vi "pulse.vi"(4 "error in":errorcluster, 5 "dwell after":u32, 6 "time on":u32, 7 "lines 2":tag) -> (0 "error out":errorcluster)   [LabVIEW 2012]
panel:
  in  "stop":bool
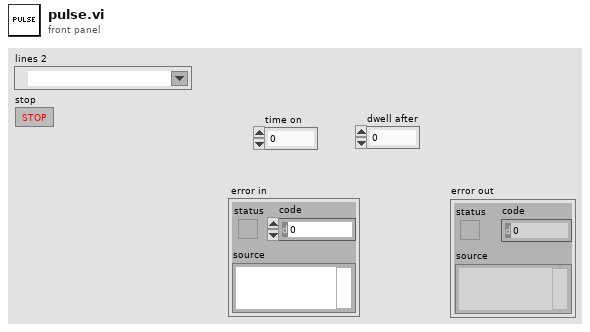
[diagram p1: front panel]
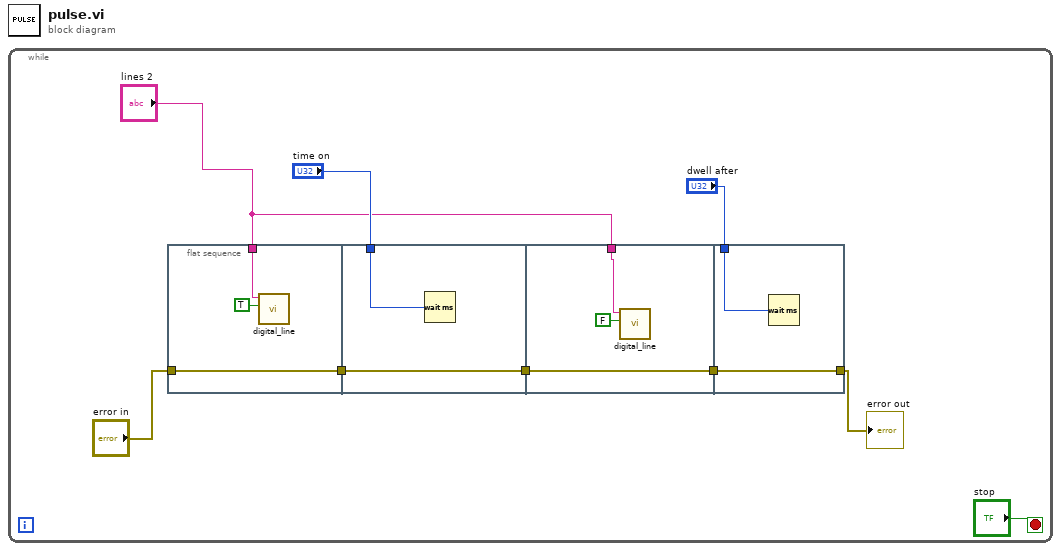
[diagram p0: block diagram]
diagram:
  n1 = while {
    stop <- "stop" stop-if-true
    n2 = flat-sequence {
      tunnel: "error in" -> [w11]
      tunnel: [w11] -> w9
      tunnel: "lines 2" -> [w10]
      tunnel: "time on" -> [w14]
      tunnel: w9 -> [w13]
      tunnel: [w13] -> w8
      tunnel: w8 -> [w17]
      tunnel: "lines 2" -> [w15]
      tunnel: [w17] -> w7
      tunnel: [w19] -> w4
      tunnel: w7 -> [w19]
      tunnel: "dwell after" -> [w18]
      frame #0 {
        n3 = call "digital_line.vi"("Boolean"=TRUE ("NewVal"), "lines"=w10) -> ()  [unwired: 5 in, 1 out]
      }
      frame #1 {
        n4 = Wait (ms)(milliseconds to wait=w14) -> ()  [unwired: 1 out]
      }
      frame #2 {
        n5 = call "digital_line.vi"("Boolean"=FALSE ("NewVal"), "lines"=w15) -> ()  [unwired: 5 in, 1 out]
      }
      frame #3 {
        n6 = Wait (ms)(milliseconds to wait=w18) -> ()  [unwired: 1 out]
      }
    }
    "error out" <- w4
  }
